vi "Randomize Starts.vi"(8 "error in (no error)":errorcluster, 11 "Game in":refnum<class "Game.lvclass">) -> (0 "error out":errorcluster, 3 "Game out":refnum<class "Game.lvclass">)   [LabVIEW 2020, in "SquareBattle.lvlib" / "Game.lvclass"]
uses:
  Game.lvclass
  Game.lvclass/Game.ctl
  Map/Map.lvclass
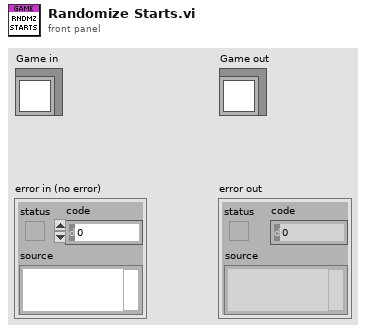
[diagram p1: front panel]
types:
  T1 = typedef "SquareBattle.lvlib/Position.ctl" = cluster{"Row":i32, "Col":i32}
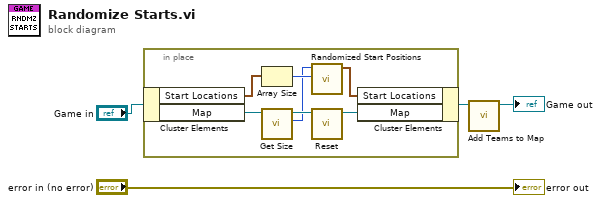
[diagram p0: block diagram]
diagram:
  n1 = in-place {
    n2 = in-place-cluster #1("Game in") -> ("Start Locations"=w8:T1[], "Map"=w11:refnum<class "Map.lvclass">)
    n3 = Array Size(array=w8) -> (size(s)=w7:i32)
    n4 = call "Get Size.vi"("Map in"=w11) -> ("Size"=w6:i32, "Map out"=w10:refnum<class "Map.lvclass">)  [unwired: 9 in]
    n5 = call "Randomized Start Positions.vi"("Player Count"=w7, "Size"=w6) -> ("Positions"=w5:T1[])  [unwired: 9 in]
    n6 = call "Reset.vi"("Map in"=w10) -> ("Map out"=w9:refnum<class "Map.lvclass">)  [unwired: 9 in, 1 out]
    n7 = in-place-cluster #1("Start Locations"=w5, "Map"=w9) -> (w2:refnum<class "Game.lvclass">)
  }
  n8 = call "Add Teams to Map.vi"("Game in"=w2) -> ("Game out"=→"Game out":refnum<class "Game.lvclass">)  [unwired: 10 in]
  "error out" <- "error in (no error)"
